vi "Actor Core.vi"(8 "error in":errorcluster, 11 "Measure-Pulse in":refnum<class "LabActor.lvclass">) -> (0 "error out":errorcluster, 3 "Actor out":refnum<class "Actor.lvclass">)   [LabVIEW 2016, in "LabActor.lvclass"]
doc: "(<B>Filename</B>: Actor Framework.lvlib:Actor.lvclass:Actor Core.vi)\n\nReceives messages to the actor, reacts to them, and initiates any error handling that may shut the actor down.\n\nDescendant classes may override this VI to append parallel tasks for the actor to complete while it handles messages. Overrides use the Call Parent Method node."
uses:
  LabActor.lvclass
  C:/github/LabActor/Controllers/Application Controller/Application Controller.lvclass
  C:/github/LabActor/Template Module/Template Module.lvclass
  C:/Program Files/National Instruments/LabVIEW 2016/vi.lib/ActorFramework/Actor/Actor.lvclass
  <vilib>/ActorFramework/Actor/Actor.lvclass
  NHMFL_Core/Libraries/Queued Listbox/Queued Listbox.xctl
  LabActor.lvclass/LabActor.ctl
  Controllers/Application Controller/Application Controller.lvclass/Application Controller.ctl
  Template Module/Template Module.lvclass/Template Module.ctl
  <vilib>/ActorFramework/Actor/Actor.lvclass/Actor.ctl
  <vilib>/ActorFramework/Message Enqueuer/Message Enqueuer.lvclass/Message Enqueuer.ctl
  Controllers/Application Controller Messages/Pulse Acquired Result/Pulse Acquired Result.lvclass
  C:/github/LabActor/Template Module Messages/Result Reply Msg/Result Reply Msg.lvclass
  Controllers/Application Controller Messages/Pulse Acquired Result/Pulse Acquired Result.lvclass/Pulse Acquired Result.ctl
  LabActor Messages/Start Pulse Measurements Msg/Start Measurements Command Msg.lvclass/Start Measurements Command Msg.ctl
  LabActor Messages/Stop Measurements Command Msg/Stop Measurements Command Msg.lvclass/Stop Measurements Command Msg.ctl
  Worker Messages/Pause Work Msg/Pause Work Msg.lvclass
  C:/Program Files/National Instruments/LabVIEW 2016/vi.lib/ActorFramework/Message/Message.lvclass
  Worker Messages/Un-Pause Work Msg/Un-Pause Work Msg.lvclass
  Template Module Messages/Message Nested Object Msg/Message Nested Object Msg.lvclass/Message Nested Object Msg.ctl
  <vilib>/Utility/sysdir.llb/System Directory Type.ctl
  Template Module Messages/Save Configuration Msg/Save Configuration Msg.lvclass/Save Configuration Msg.ctl
  Template Module Messages/Open Item Msg/Open Item Msg.lvclass/Open Item Msg.ctl
  Plots/Plot types.ctl
  Controllers/Application Controller Messages/Open Waveform File Plot Msg/Open Waveform File Plot Msg.lvclass/Open Waveform File Plot Msg.ctl
  Controllers/Application Controller Messages/Pulse Acquired Result/Write Open plot.vi
  Controllers/Application Controller/Write Armed ref.vi
  Controllers/Application Controller/Write Monitor Running.vi
  Controllers/Application Controller/Write Monitor ref.vi
  Controllers/Application Controller/Write Postproc ref.vi
  Template Module/Read stop event.vi
  Template Module/Read Open item event.vi
  <vilib>/ActorFramework/Message Enqueuer/Init from Existing Queue.vi
  <vilib>/ActorFramework/Message Enqueuer/Enqueue.vi
  <vilib>/ActorFramework/Stop Msg/Stop Msg.lvclass
  LabActor Messages/Start Pulse Measurements Msg/Start Measurements Command Msg.lvclass
  LabActor Messages/Stop Measurements Command Msg/Stop Measurements Command Msg.lvclass
  Template Module Messages/Message Nested Object Msg/Message Nested Object Msg.lvclass
  Template Module Messages/Save Configuration Msg/Save Configuration Msg.lvclass
  Template Module Messages/Open Item Msg/Open Item Msg.lvclass
  Controllers/Application Controller Messages/Open Waveform File Plot Msg/Open Waveform File Plot Msg.lvclass
  <vilib>/ActorFramework/Message Priority Queue/Priority Enqueue.vi
  Controllers/Application Controller/Application Controller.lvclass
  <vilib>/ActorFramework/Message Enqueuer/Message Enqueuer.lvclass
  Template Module Messages/Restore Configuration Msg/Restore Configuration Msg.lvclass
panel:
  in  "About Button":bool
  in  "Pause":bool
  in  "Disarm":bool
  in  "Clear log":bool
  out "Error log":string
  in  "Full XY Plot":bool
  out "Monitor file":path caption="Monintor\nFile"
  in  "View Waveform":bool
  out "PEAK FIELD":dbl format="%#.2g"
  in  "Exit":bool
  in  "Monitor configuration":bool
  in  "Pulse configuration":bool
  in  "Refresh Button":bool
  out "Pulse file":path caption="Pulse\nFile"
  in  "Write cfg":bool
  in  "Read cfg":bool
  in  "View XY Plot":bool
  out "Monitor Running":bool
  out "Armed":bool
  in  "Arm":bool
  in  "Stop monitor":bool
  in  "Start monitor":bool
  in  "Monitor":string[](xcontrol)
  in  "Process Pulse":string[](xcontrol)
  in  "Acquire Pulse":string[](xcontrol)
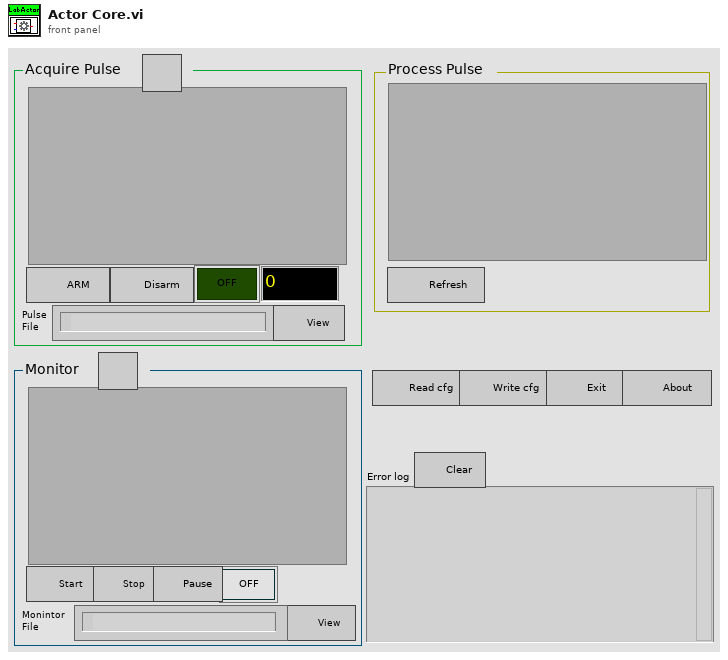
[diagram p1: front panel]
types:
  T1 = typedef "Plot types.ctl" = enum16{"Waveform Plot", "XY Plot", "Full XY"}
  T2 = typedef "System Directory Type.ctl" = i32
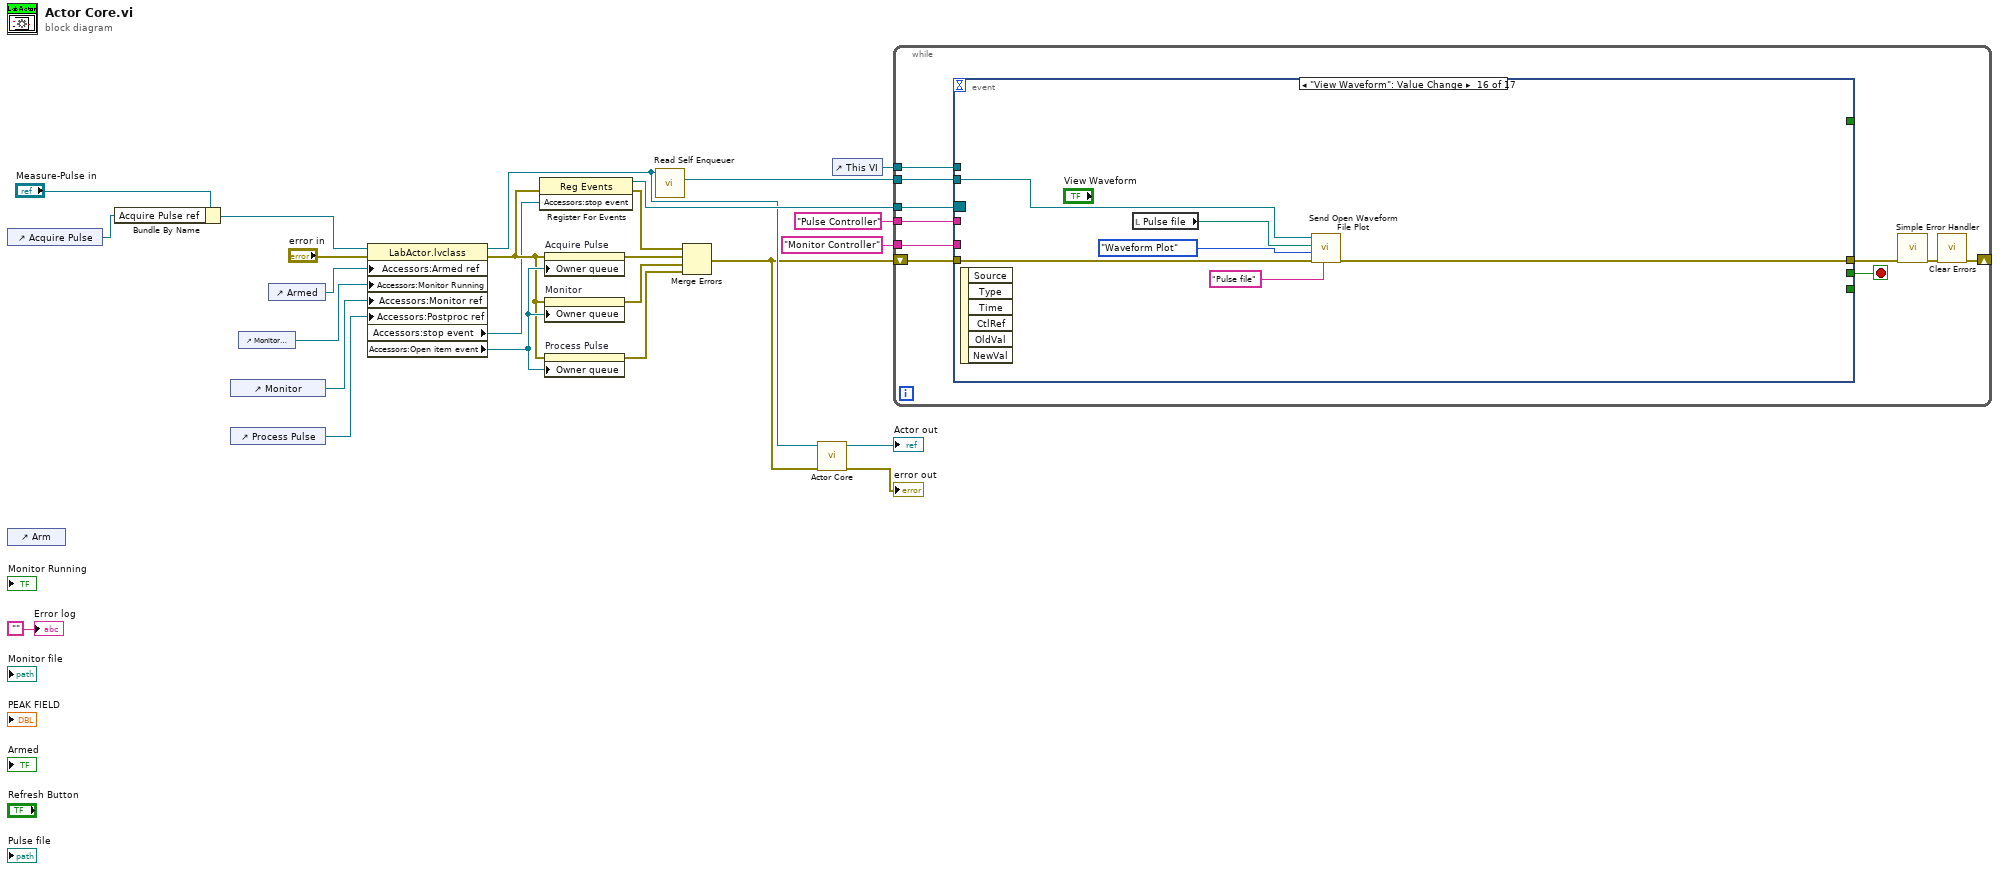
[diagram p0: block diagram]
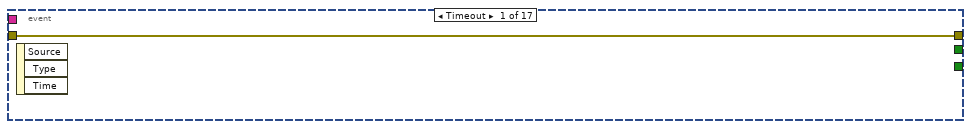
[diagram p2: hidden frame]
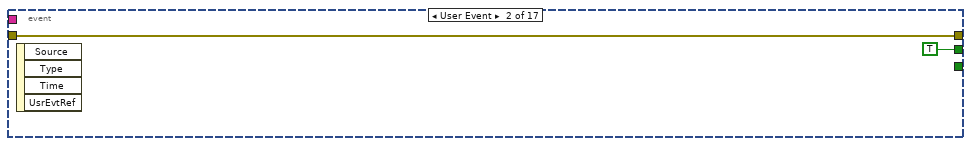
[diagram p3: hidden frame]
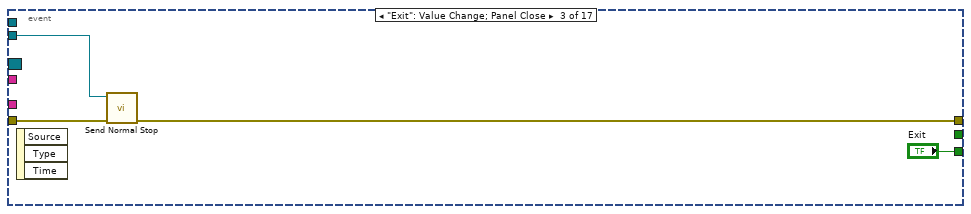
[diagram p4: hidden frame]
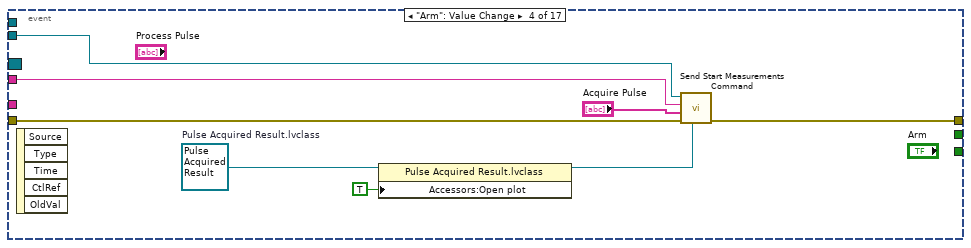
[diagram p5: hidden frame]
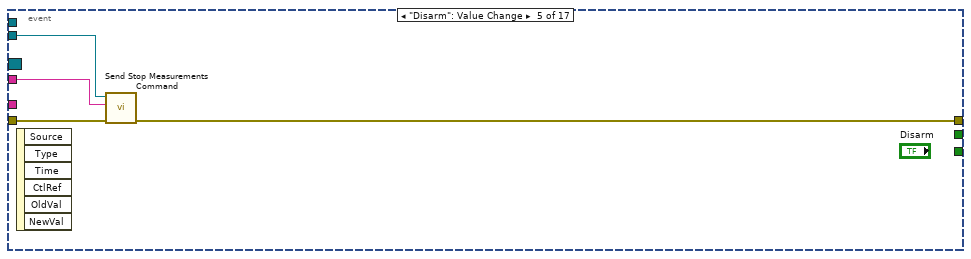
[diagram p6: hidden frame]
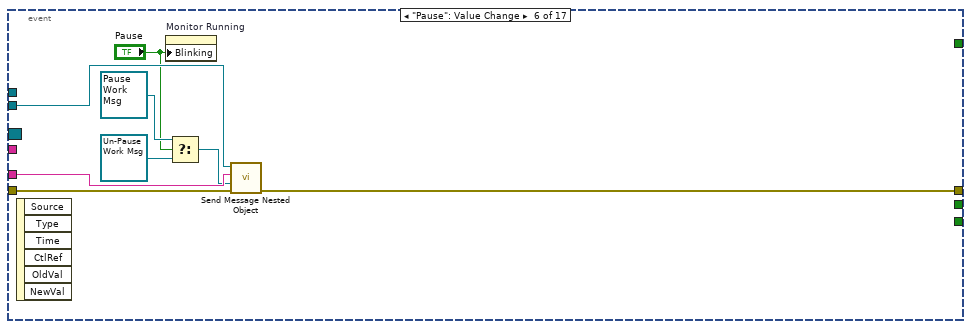
[diagram p7: hidden frame]
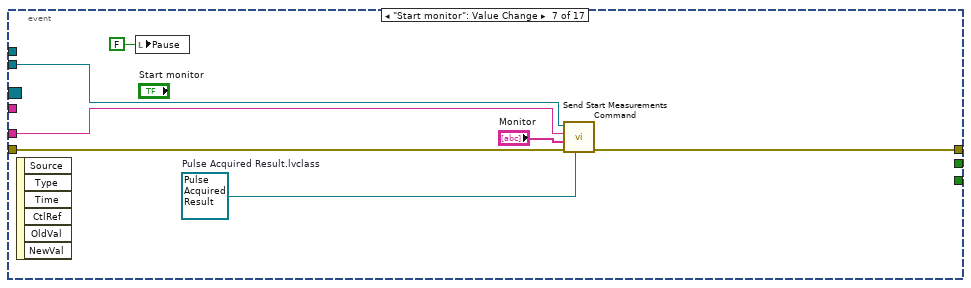
[diagram p8: hidden frame]
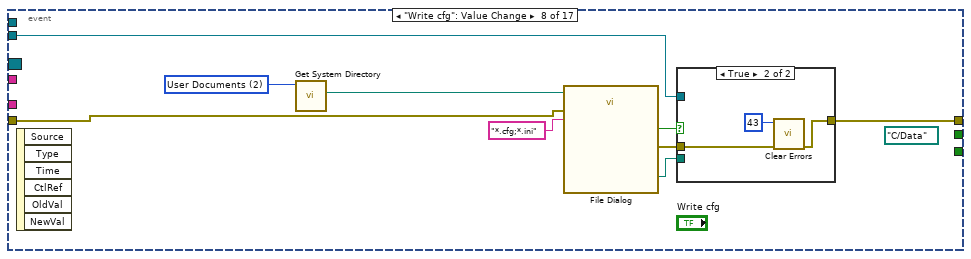
[diagram p9: hidden frame]
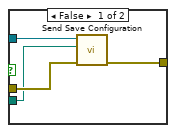
[diagram p10: hidden frame]
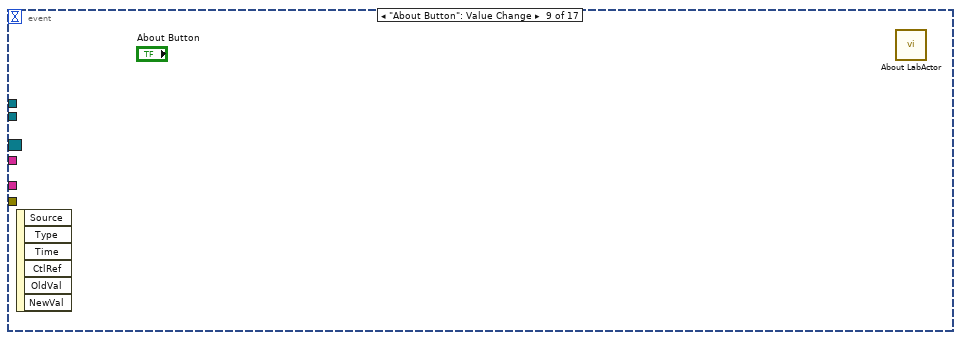
[diagram p11: hidden frame]
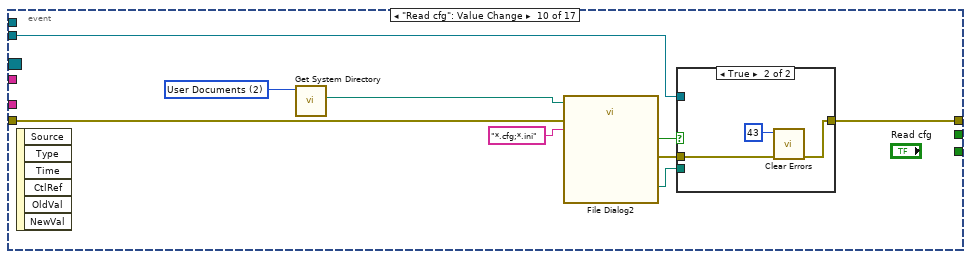
[diagram p12: hidden frame]
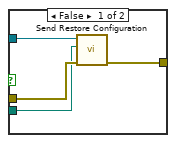
[diagram p13: hidden frame]
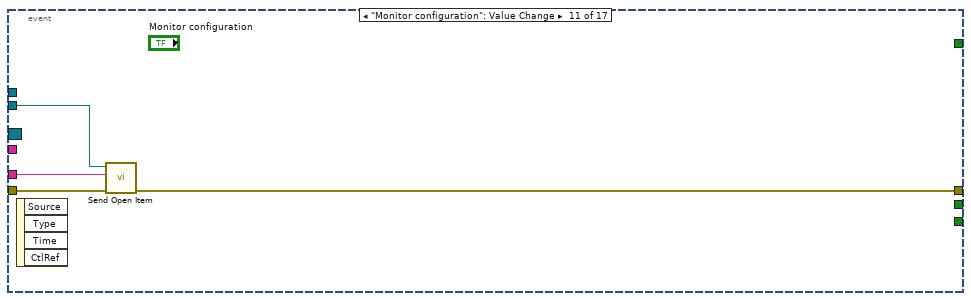
[diagram p14: hidden frame]
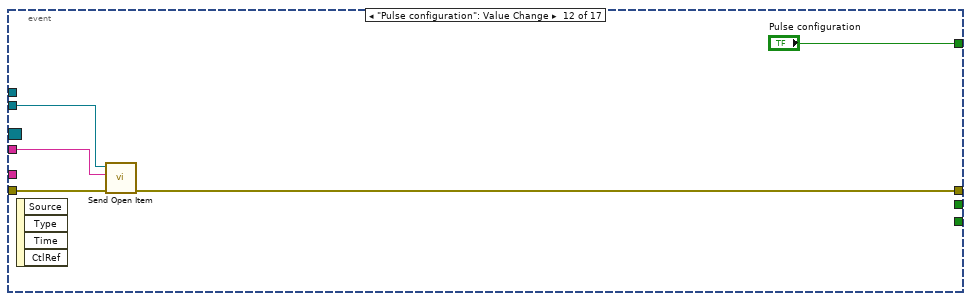
[diagram p15: hidden frame]
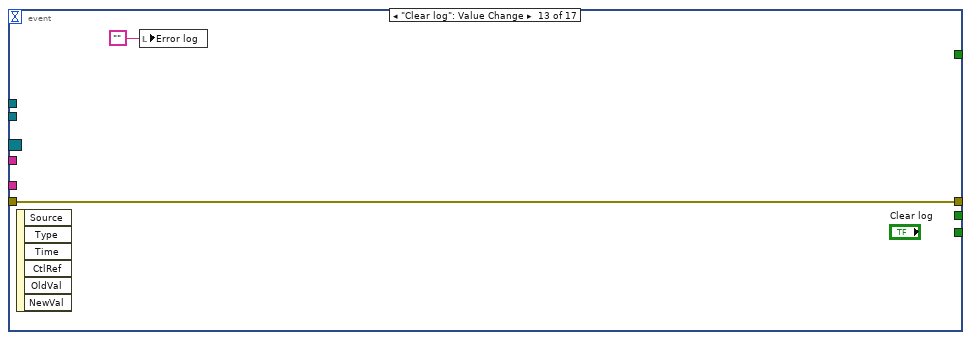
[diagram p16: hidden frame]
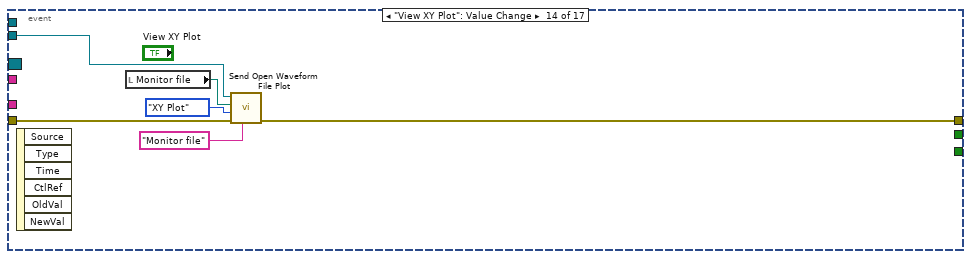
[diagram p17: hidden frame]
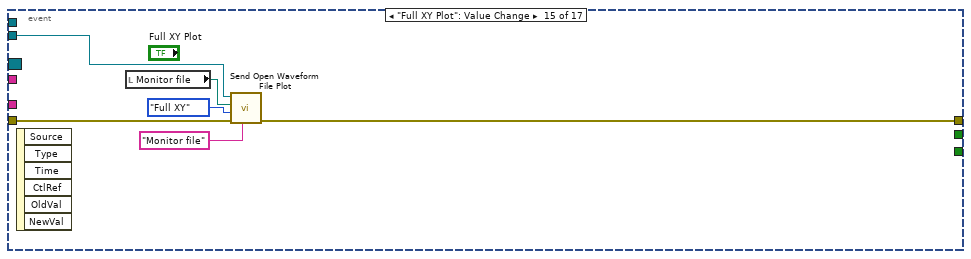
[diagram p18: hidden frame]
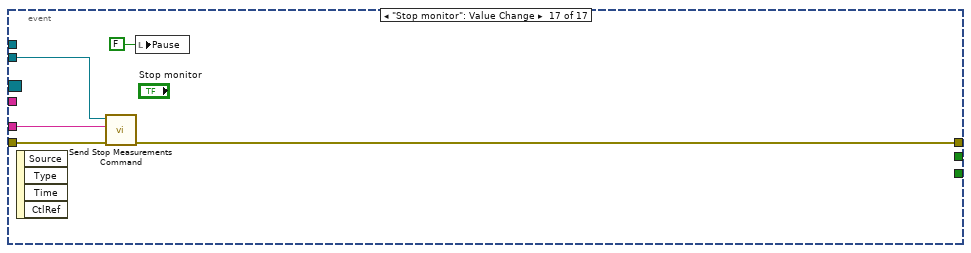
[diagram p19: hidden frame]
diagram:
  n1 = control-ref of="Acquire Pulse"() -> (w12:refnum<vi>)
  n2 = control-ref of="Arm"() -> ()  [unwired: 1 out]
  n3 = Bundle By Name(cluster="Measure-Pulse in", "Acquire Pulse ref"=w12) -> (w2:refnum<class "LabActor.lvclass">)
  n4 = control-ref of="Monitor"() -> (w5:refnum<vi>)
  n5 = control-ref of="Process Pulse"() -> (w4:refnum<vi>)
  n6 = control-ref of="Monitor Running"() -> (w6:refnum<vi>)
  n7 = control-ref of="Armed"() -> (w7:refnum<vi>)
  n8 = property class="LabActor.lvclass"(reference=w2, error in="error in", "Accessors:Armed ref"=w7, "Accessors:Monitor Running"=w6, "Accessors:Monitor ref"=w5, "Accessors:Postproc ref"=w4) -> (reference out=w14:refnum<class "LabActor.lvclass">, error out=w17:errorcluster, "Accessors:stop event"=w8:refnum<user-event>, "Accessors:Open item event"=w21:refnum<user-event>)
  n9 = register-events(error in=w17, w8) -> (reference out=w22:refnum<event-registration>, error out=w16:errorcluster)  [unwired: 1 in]
  n10 = property on="Acquire Pulse" class="Queued Listbox (strict)"(error in=w17, "Owner queue"=w21) -> (error out=w20:errorcluster)  [unwired: 1 in, 1 out]
  n11 = property on="Monitor" class="Queued Listbox (strict)"(error in=w17, "Owner queue"=w21) -> (error out=w19:errorcluster)  [unwired: 1 in, 1 out]
  n12 = property on="Process Pulse" class="Queued Listbox (strict)"(error in=w17, "Owner queue"=w21) -> (error out=w18:errorcluster)  [unwired: 1 in, 1 out]
  n13 = call <vilib>:"Read Self Enqueuer.vi"("Actor"=w14) -> ("Self Enqueuer"=w13:refnum<class "Message Enqueuer.lvclass">)  [unwired: 10 in]
  n14 = Merge Errors(w16, w20, w19, w18) -> (w3:errorcluster)
  n15 = call-parent "Actor Core.vi"("error in"=w3, "Measure Object in"=w14) -> ("error out"=→"error out":errorcluster, "Actor out"=→"Actor out":refnum<class "Actor.lvclass">)  [unwired: 8 in]
  n16 = control-ref of="This VI"() -> (w1:refnum<vi>)
  n17 = while {
    tunnel: w22 -> [w35]
    tunnel: w13 -> [w33]
    tunnel: "Monitor Controller" ("Controller name") -> [w32]
    tunnel: "Pulse Controller" ("Item name") -> [w31]
    shift-right: [w27] -> _
    shift-left: w3 -> [w30]
    tunnel: w1 -> [w26]
    stop <- w34 stop-if-true
    n18 = event shown="[15] \"View Waveform\": Value Change" {
      selector: w35 -> [_ _ _ _ _ _ _ _ _ _ _ _ _ _ _ _ _]
      dyn-events: _ -> [_ _ _ _ _ _ _ _ _ _ _ _ _ _ _ _ _]
      timeout: _ -> [_ _ _ _ _ _ _ _ _ _ _ _ _ _ _ _ _]
      tunnel: [_ TRUE _ _ _ _ _ _ _ _ _ _ _ _ _ _ _] -> w34
      tunnel: w33 -> [_ _ w41 w45 w54 w58 w68 w75 _ w89 w105 w109 _ w118 w124 w129 w135]
      tunnel: [_ _ _ _ _ _ _ _ _ _ _ "Pulse configuration" _ _ _ _ _] -> _
      tunnel: [_ _ "Exit" _ _ _ _ _ _ _ _ _ _ _ _ _ _] -> _
      tunnel: w32 -> [_ _ _ _ _ w62 w67 _ _ _ w104 _ _ _ _ _ w134]
      tunnel: w31 -> [_ _ _ w49 w53 _ _ _ _ _ _ w108 _ _ _ _ _]
      tunnel: w30 -> [w36 w37 w40 w44 w52 w56 w64 w71 _ w87 w103 w107 w111 w114 w120 w126 w132]
      tunnel: [w36 w37 w39 w43 w51 w55 w63 w70 _ w86 w102 w106 w111 w113 w119 w125 w131] -> w29
      tunnel: w26 -> [_ _ _ _ _ _ _ _ _ _ _ _ _ _ _ _ _]
      event Timeout {
        n19 = event-data() -> ()  [unwired: 1 in, 3 out]
      }
      event User Event {
        n20 = event-data() -> ()  [unwired: 1 in, 4 out]
      }
      event "Exit": Value Change; Panel Close {
        n21 = event-data() -> ()  [unwired: 1 in, 3 out]
        n22 = call <vilib>:"Send Normal Stop.vi"("error in (no error)"=w40, "Message Enqueuer"=w41) -> ("error out"=w39:errorcluster)  [unwired: 9 in]
      }
      event "Arm": Value Change {
        w48 = refnum<class "Pulse Acquired Result.lvclass"> refnum  # Pulse Acquired Result.lvclass
        n23 = event-data() -> ()  [unwired: 1 in, 5 out]
        n24 = property class="Pulse Acquired Result.lvclass"(reference=w48, "Accessors:Open plot"=TRUE ("Open plot")) -> (reference out=w47:refnum<class "Pulse Acquired Result.lvclass">)  [unwired: 1 in, 1 out]
        n25 = call "Send Start Measurements Command.vi"("Reply to me"=w47, "error in (no error)"=w44, "Objects"="Acquire Pulse", "Controller name"=w49, "Message Enqueuer"=w45) -> ("error out"=w43:errorcluster)  [unwired: 5 in, 1 out]
      }
      event "Disarm": Value Change {
        n26 = event-data() -> ()  [unwired: 1 in, 6 out]
        n27 = call "Send Stop Measurements Command.vi"("error in (no error)"=w52, "Measurement Controller"=w53, "Message Enqueuer"=w54) -> ("error out"=w51:errorcluster)  [unwired: 7 in, 1 out]
      }
      event "Pause": Value Change {
        n28 = event-data() -> ()  [unwired: 1 in, 6 out]
        n29 = property on="Monitor Running" class="Bool (strict)"("Blinking"="Pause") -> ()  [unwired: 2 in, 2 out]
        n30 = Select(t=refnum<class "Pause Work Msg.lvclass"> refnum ("Pause Work Msg.lvclass"), s="Pause", f=refnum<class "Un-Pause Work Msg.lvclass"> refnum ("Un-Pause Work Msg.lvclass")) -> (s? t:f=w59:refnum<class "Message.lvclass">)
        n31 = call "Send Message Nested Object.vi"("error in (no error)"=w56, "Message"=w59, "Name"=w62, "Message Enqueuer"=w58) -> ("error out"=w55:errorcluster)  [unwired: 6 in, 1 out]
      }
      event "Start monitor": Value Change {
        w66 = refnum<class "Pulse Acquired Result.lvclass"> refnum  # Pulse Acquired Result.lvclass
        n32 = event-data() -> ()  [unwired: 1 in, 6 out]
        n33 = local write "Pause"(FALSE ("Pause")) -> ()
        n34 = call "Send Start Measurements Command.vi"("Reply to me"=w66, "error in (no error)"=w64, "Objects"="Monitor", "Controller name"=w67, "Message Enqueuer"=w68) -> ("error out"=w63:errorcluster)  [unwired: 5 in, 1 out]
      }
      event "Write cfg": Value Change {
        w73 = T2 2 items=["User Home"=0, "User Desktop"=1, "User Documents"=2, "User Application Data"=3, "User Preferences"=4, "User Temporary"=5, "Public Documents"=6, "Public Application Data"=7, "Public Preferences"=8, "Public Cache"=13, "System Core Libraries"=9, "System Installed Libraries"=10, "Application Files"=11, "Boot Volume Root"=12] ("system directory type")
        (unwired) path "C:/Data" ("start path")
        n35 = event-data() -> ()  [unwired: 1 in, 6 out]
        n36 = call <vilib>:"Get System Directory.vi"("system directory type"=w73) -> ("system directory"=w72:path)  [unwired: 10 in]
        n37 = call "File Dialog"("start path"=w72, "error in"=w71, "pattern (all files)"="*.cfg;*.ini") -> ("selected path"=w77:path, "cancelled"=w78:bool, "error out"=w74:errorcluster)  [unwired: 9 in, 1 out]
        n38 = case shown="True" w78 {
          tunnel: w77 -> [w80 _]
          tunnel: w75 -> [w82 _]
          tunnel: w74 -> [w81 w85]
          tunnel: [w79 w84] -> w70
          frame False {
            n39 = call "Send Save Configuration.vi"("error in (no error)"=w81, "File path"=w80, "Message Enqueuer"=w82) -> ("error out"=w79:errorcluster)  [unwired: 7 in, 1 out]
          }
          frame True {
            n40 = call <vilib>:"Clear Errors.vi"("error in (no error)"=w85, "specific error code to clear (0: all)"=43) -> ("error out"=w84:errorcluster)  [unwired: 4 in, 1 out]
          }
        }
      }
      event "About Button": Value Change {
        n41 = event-data() -> ()  [unwired: 1 in, 6 out]
        n42 = call "About LabActor.vi"() -> ()  [unwired: 12 in]
      }
      event "Read cfg": Value Change {
        w91 = T2 2 items=["User Home"=0, "User Desktop"=1, "User Documents"=2, "User Application Data"=3, "User Preferences"=4, "User Temporary"=5, "Public Documents"=6, "Public Application Data"=7, "Public Preferences"=8, "Public Cache"=13, "System Core Libraries"=9, "System Installed Libraries"=10, "Application Files"=11, "Boot Volume Root"=12] ("system directory type")
        n43 = event-data() -> ()  [unwired: 1 in, 6 out]
        n44 = call <vilib>:"Get System Directory.vi"("system directory type"=w91) -> ("system directory"=w90:path)  [unwired: 10 in]
        n45 = call "File Dialog2"("start path"=w90, "error in"=w87, "pattern (all files)"="*.cfg;*.ini") -> ("selected path"=w94:path, "cancelled"=w88:bool, "error out"=w92:errorcluster)  [unwired: 9 in, 1 out]
        n46 = case shown="True" w88 {
          tunnel: w94 -> [w96 _]
          tunnel: w89 -> [w98 _]
          tunnel: w92 -> [w97 w101]
          tunnel: [w95 w100] -> w86
          frame False {
            n47 = call "Send Restore Configuration.vi"("error in (no error)"=w97, "File path"=w96, "Message Enqueuer"=w98) -> ("error out"=w95:errorcluster)  [unwired: 7 in, 1 out]
          }
          frame True {
            n48 = call <vilib>:"Clear Errors.vi"("error in (no error)"=w101, "specific error code to clear (0: all)"=43) -> ("error out"=w100:errorcluster)  [unwired: 4 in, 1 out]
          }
        }
      }
      event "Monitor configuration": Value Change {
        n49 = event-data() -> ()  [unwired: 1 in, 4 out]
        n50 = call "Send Open Item.vi"("error in (no error)"=w103, "Item name"=w104, "Message Enqueuer"=w105) -> ("error out"=w102:errorcluster)  [unwired: 7 in, 1 out]
      }
      event "Pulse configuration": Value Change {
        n51 = event-data() -> ()  [unwired: 1 in, 4 out]
        n52 = call "Send Open Item.vi"("error in (no error)"=w107, "Item name"=w108, "Message Enqueuer"=w109) -> ("error out"=w106:errorcluster)  [unwired: 7 in, 1 out]
      }
      event "Clear log": Value Change {
        n53 = event-data() -> ()  [unwired: 1 in, 6 out]
        n54 = local write "Error log"("" ("Error log")) -> ()
      }
      event "View XY Plot": Value Change {
        n55 = event-data() -> ()  [unwired: 1 in, 6 out]
        n56 = local read "Monitor file"() -> (w117:path)
        n57 = call "Send Open Waveform File Plot.vi"("Plot group"="Monitor file" ("Control Name"), "error in (no error)"=w114, "Plot type"=Plot_types."XY Plot", "File Path Control"=w117, "Message Enqueuer"=w118) -> ("error out"=w113:errorcluster)  [unwired: 5 in, 1 out]
      }
      event "Full XY Plot": Value Change {
        n58 = event-data() -> ()  [unwired: 1 in, 6 out]
        n59 = local read "Monitor file"() -> (w123:path)
        n60 = call "Send Open Waveform File Plot.vi"("Plot group"="Monitor file" ("Control Name"), "error in (no error)"=w120, "Plot type"=Plot_types."Full XY", "File Path Control"=w123, "Message Enqueuer"=w124) -> ("error out"=w119:errorcluster)  [unwired: 5 in, 1 out]
      }
      event "View Waveform": Value Change {
        n61 = event-data() -> ()  [unwired: 1 in, 6 out]
        n62 = local read "Pulse file"() -> (w128:path)
        n63 = call "Send Open Waveform File Plot.vi"("Plot group"="Pulse file" ("Control Name"), "error in (no error)"=w126, "Plot type"=Plot_types."Waveform Plot", "File Path Control"=w128, "Message Enqueuer"=w129) -> ("error out"=w125:errorcluster)  [unwired: 5 in, 1 out]
      }
      event "Stop monitor": Value Change {
        n64 = event-data() -> ()  [unwired: 1 in, 4 out]
        n65 = call "Send Stop Measurements Command.vi"("error in (no error)"=w132, "Measurement Controller"=w134, "Message Enqueuer"=w135) -> ("error out"=w131:errorcluster)  [unwired: 7 in, 1 out]
        n66 = local write "Pause"(FALSE ("Pause")) -> ()
      }
    }
    n67 = call <vilib>:"Simple Error Handler.vi"("error in (no error)"=w29) -> ("error out"=w28:errorcluster)  [unwired: 4 in, 4 out]
    n68 = call <vilib>:"Clear Errors.vi"("error in (no error)"=w28) -> ("error out"=w27:errorcluster)  [unwired: 5 in, 1 out]
  }
  "Error log" <- "" ("Error log")
